vi "GetBounds.vi"(0 "Exceed RC Volcano Series in":refnum<class "Exceed RC Volcano Series.lvclass">, 11 "error in (no error)":errorcluster) -> (4 "Exceed RC Volcano Series out":refnum<class "Exceed RC Volcano Series.lvclass">, 10 "Calibrate?":bool, 12 "PWM Frequency":dbl, 13 "Duty Cycle Min":dbl, 14 "Duty Cycle Max":dbl, 15 "error out":errorcluster)   [LabVIEW 2015, in "Exceed RC Volcano Series.lvclass"]
uses:
  Exceed RC Volcano Series.lvclass
  Exceed RC Volcano Series.lvclass/Exceed RC Volcano Series.ctl
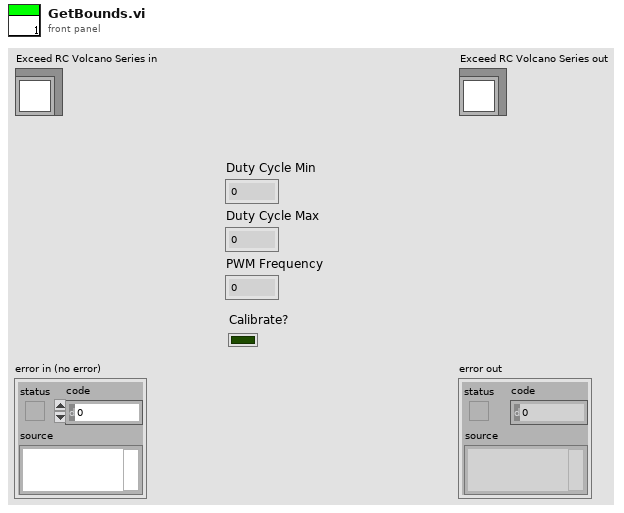
[diagram p1: front panel]
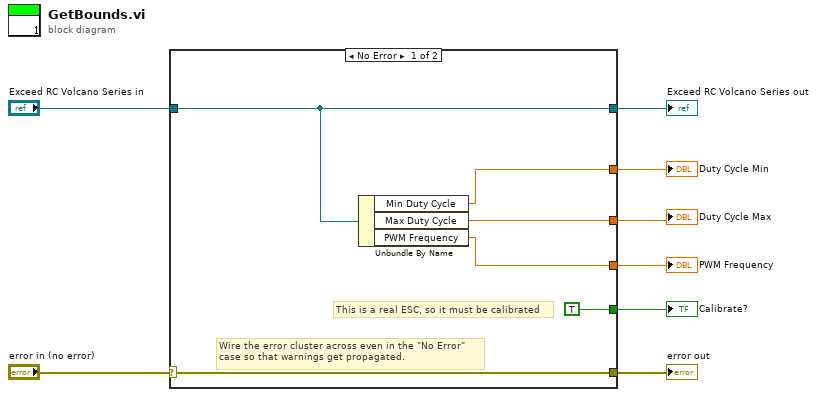
[diagram p0: block diagram]
diagram:
  n1 = case shown="No Error" "error in (no error)" {
    selector: "error in (no error)" -> [w14 w16]
    tunnel: [w14 w16] -> w7
    tunnel: [w13 w15] -> w5
    tunnel: "Exceed RC Volcano Series in" -> [w13 w15]
    tunnel: [w12 _] -> w4
    tunnel: [w11 _] -> w3
    tunnel: [w10 _] -> w2
    tunnel: [TRUE ("Calibrate?") _] -> w1
    frame No Error {
      # "This is a real ESC, so it must be calibrated"
      # "Wire the error cluster across even in the \"No Error\"\ncase so that warnings get propagated."
      n2 = Unbundle By Name(w13) -> ("Min Duty Cycle"=w12:dbl, "Max Duty Cycle"=w11:dbl, "PWM Frequency"=w10:dbl)
    }
    frame Error {
    }
  }
  "error out" <- w7
  "Exceed RC Volcano Series out" <- w5
  "Duty Cycle Min" <- w4
  "Duty Cycle Max" <- w3
  "PWM Frequency" <- w2
  "Calibrate?" <- w1
